vi "温控命令.vi"(10 "布尔":bool=TRUE, 11 "队列输入":refnum<queue>) -> ()   [LabVIEW 2016, in "PLC.lvlib"]
uses:
  PLC.lvlib
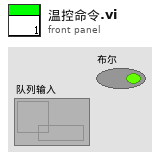
[diagram p1: front panel]
types:
  T1 = cluster{"命令":string, "data":cluster{"starting address":u16, "coil values":bool[]}}
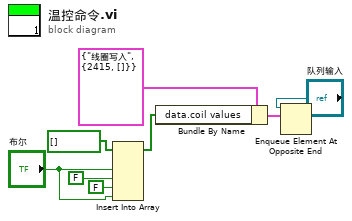
[diagram p0: block diagram]
diagram:
  n1 = Insert Into Array(array=bool[] [] ("data.coil values"), new element #1="布尔", new element #2=FALSE ("新元素/子数组"), new element #3=FALSE ("新元素/子数组"), new element #4="布尔") -> (w4:bool[])  [unwired: 1 in]
  n2 = Bundle By Name(cluster=T1 {"命令"="线圈写入", "data"={"starting address"=2415, "coil values"=[]}} ("元素"), "data.coil values"=w4) -> (w6:T1)
  n3 = Enqueue Element At Opposite End(queue="队列输入", element=w6) -> ()  [unwired: 2 in, 3 out]
